vi "SortContourCheckZero.vi"(11 "LineArray":T3[](array[typedef])) -> (3 "Polys":T1[](array[typedef]))   [LabVIEW 2014]
uses:
  TypeDefs/Line2D.ctl
  TypeDefs/Point2D.ctl
  TypeDefs/Poly2D.ctl
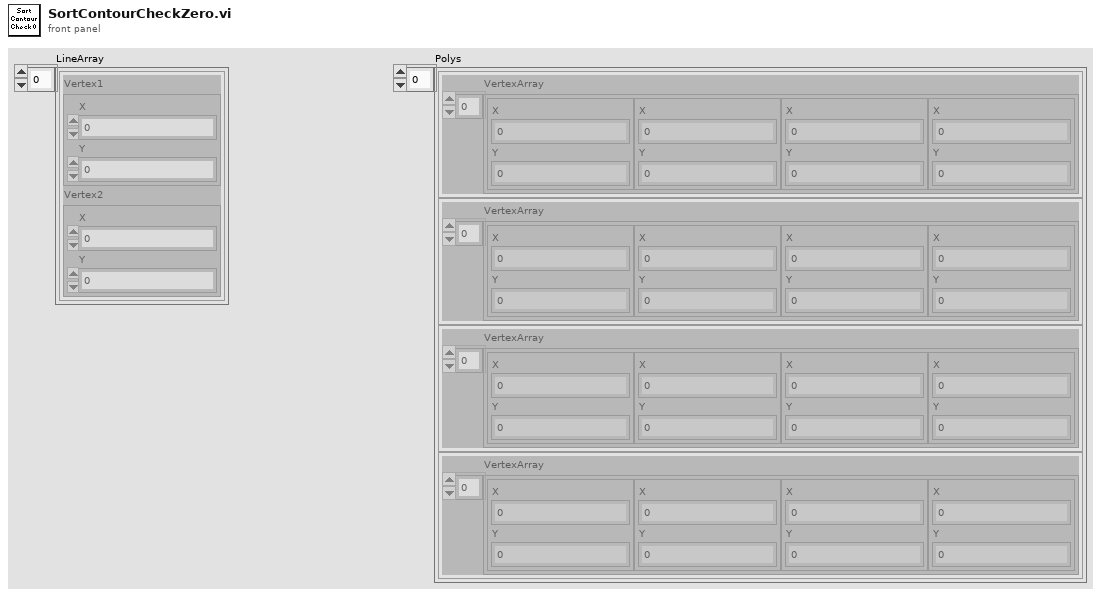
[diagram p1: front panel]
types:
  T1 = typedef "Poly2D.ctl" = cluster{"VertexArray":T2[]}
  T2 = typedef "Point2D.ctl" = cluster{"X":sgl, "Y":sgl}
  T3 = typedef "Line2D.ctl" = cluster{"Vertex1":T2, "Vertex2":T2}
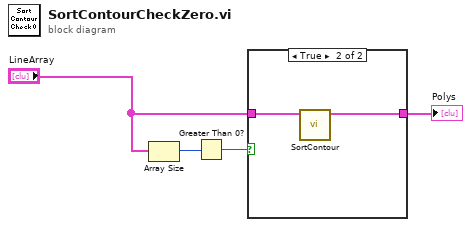
[diagram p0: block diagram]
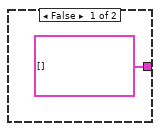
[diagram p2: hidden frame]
diagram:
  n1 = Array Size(array="LineArray") -> (size(s)=w3:i32)
  n2 = Greater Than 0?(x=w3) -> (x > 0?=w2:bool)
  n3 = case shown="True" w2 {
    tunnel: "LineArray" -> [_ w7]
    tunnel: [T1[] [] ("Polys") w6] -> w1
    frame False {
    }
    frame True {
      n4 = call "SortContour.vi"("LineArray"=w7) -> ("Polys"=w6:T1[])  [unwired: 10 in]
    }
  }
  "Polys" <- w1
